vi "Update Graphs.vi"(8 "error in (no error)":errorcluster, 11 "MFC in":refnum<class "MFC.lvclass">) -> (0 "error out":errorcluster, 3 "MFC out":refnum<class "MFC.lvclass">)   [LabVIEW 2013, in "MFC.LVLIB" / "MFC.lvclass"]
uses:
  MFC.lvclass
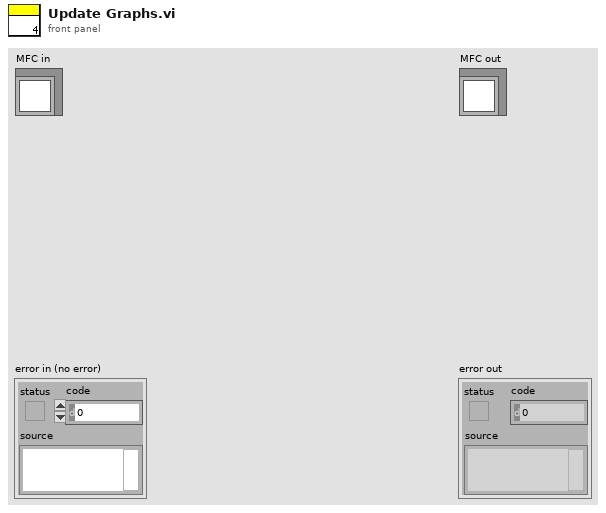
[diagram p1: front panel]
types:
  T1 = cluster{"output array":dbl[], "output array":dbl[]}
  T2 = cluster{"output array":dbl[], "output array":dbl[]}[]
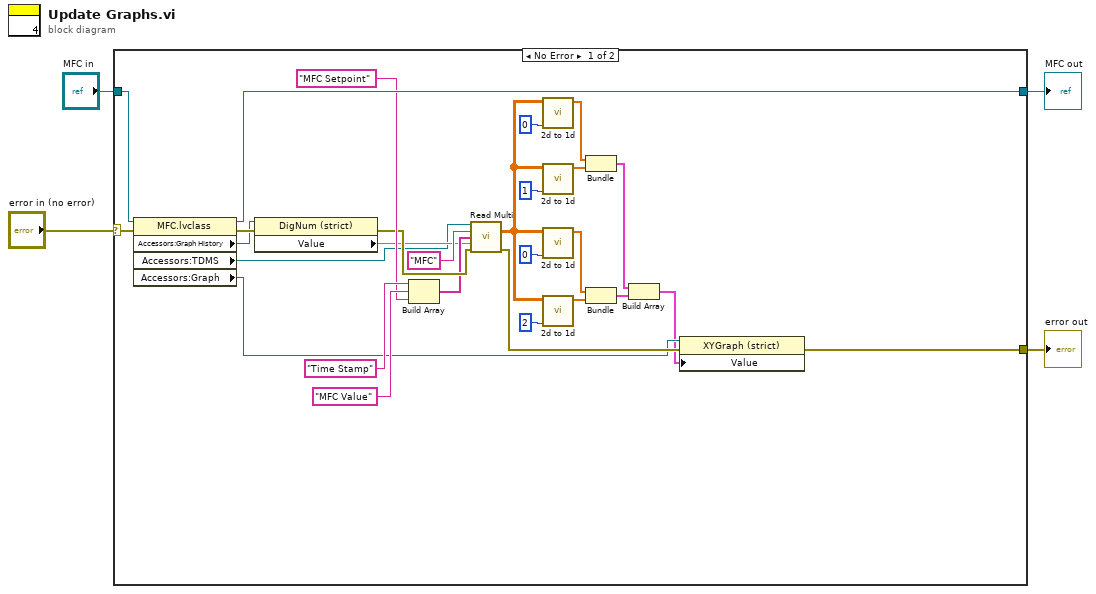
[diagram p0: block diagram]
diagram:
  n1 = case shown="No Error" "error in (no error)" {
    selector: "error in (no error)" -> [w27 w34]
    tunnel: [w5 w34] -> w1
    tunnel: [w31 w33] -> w2
    tunnel: "MFC in" -> [w32 w33]
    frame No Error {
      n2 = property class="MFC.lvclass"(reference=w32, error in=w27) -> (reference out=w31:refnum<class "MFC.lvclass">, error out=w26:errorcluster, "Accessors:Graph History"=w20:refnum<vi>, "Accessors:TDMS"=w21:refnum<k34>, "Accessors:Graph"=w18:refnum<vi>)
      n3 = property class="DigNum (strict)"(reference=w20, error in=w26) -> (error out=w25:errorcluster, "Value"=w22:dbl)  [unwired: 1 out]
      n4 = Build Array("Time Stamp" ("Channel"), "MFC Value" ("string"), "MFC Setpoint" ("string")) -> (w23:string[])
      n5 = call "Read Multi.vi"("tdms file in"=w21, "group"="MFC", "Channel"=w23, "Numeric"=w22, "error in (no error)"=w25) -> ("Array"=w7:dbl[][], "error out"=w19:errorcluster)  [unwired: 7 in, 2 out]
      n6 = call "2d to 1d.vi"("index"=0, "array"=w7) -> ("output array"=w10:dbl[])  [unwired: 9 in]
      n7 = call "2d to 1d.vi"("index"=1, "array"=w7) -> ("output array"=w11:dbl[])  [unwired: 9 in]
      n8 = call "2d to 1d.vi"("index"=0, "array"=w7) -> ("output array"=w12:dbl[])  [unwired: 9 in]
      n9 = call "2d to 1d.vi"("index"=2, "array"=w7) -> ("output array"=w13:dbl[])  [unwired: 9 in]
      n10 = Bundle("output array"=w10, "output array"=w11) -> (w9:T1)  [unwired: 1 in]
      n11 = Bundle("output array"=w12, "output array"=w13) -> (w8:T1)  [unwired: 1 in]
      n12 = Build Array(w9, w8) -> (w6:T2)
      n13 = property class="XYGraph (strict)"(reference=w18, error in=w19, "Value"=w6) -> (error out=w5:errorcluster)  [unwired: 1 out]
    }
    frame Error {
    }
  }
  "error out" <- w1
  "MFC out" <- w2
